vi "EX 2.vi"() -> ()   [LabVIEW 2018]
panel:
  out "Led":bool
  in  "Bouton 3":i32(knob) scale=0.0..10.0
  in  "Bouton 2":i32(knob) scale=0.0..10.0
  in  "Bouton 1":i32(knob) scale=0.0..10.0
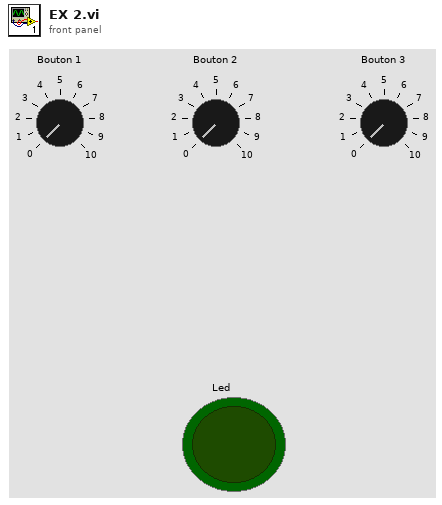
[diagram p1: front panel]
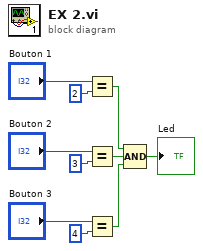
[diagram p0: block diagram]
diagram:
  n1 = Equal?(x="Bouton 1", y=2) -> (x = y?=w4:bool)
  n2 = Equal?(x="Bouton 2", y=3) -> (x = y?=w3:bool)
  n3 = Equal?(x="Bouton 3", y=4) -> (x = y?=w2:bool)
  n4 = Compound Arithmetic op=AND(w4, w3, w2) -> (→"Led":bool)
